vi "Display_Bad_Positions.vi"() -> ()   [LabVIEW 2022 SP3]
uses:
  Collision_Detection/Triangles/EnFlo specific/Collision Mode.ctl
  Collision_Detection/Triangles/EnFlo specific/Collision Detection global.vi
panel:
  out "Error Comments":string
  in  "Show Red Collision Sphere":bool=TRUE
  in  "Display Line Number":i32=1 min=1
  out "Table Control":string[][](table)
  in  "Choose Bad Point file":path
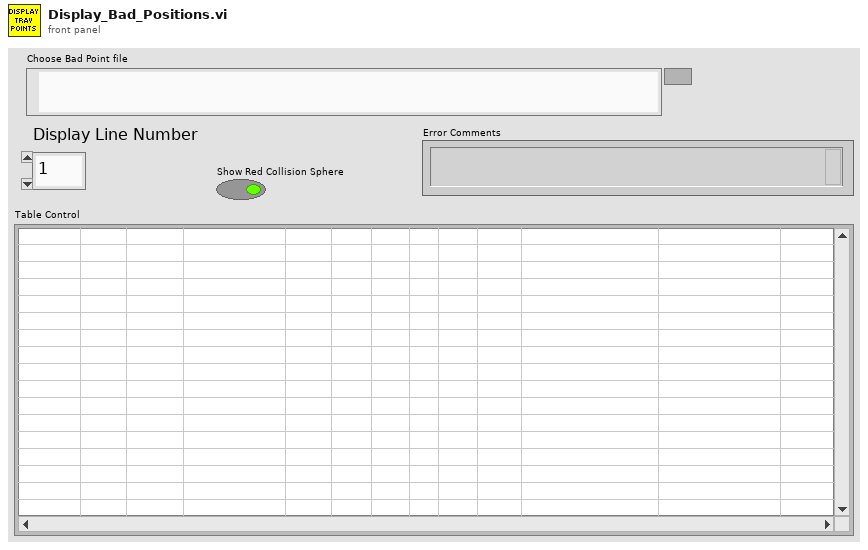
[diagram p1: front panel]
types:
  T1 = typedef "Collision Mode.ctl" = enum16{"Traverse - Tunnel", "Traverse - Model", "Traverse - Fixed objects", "Traverse - Traverse", "Traverse - All"}
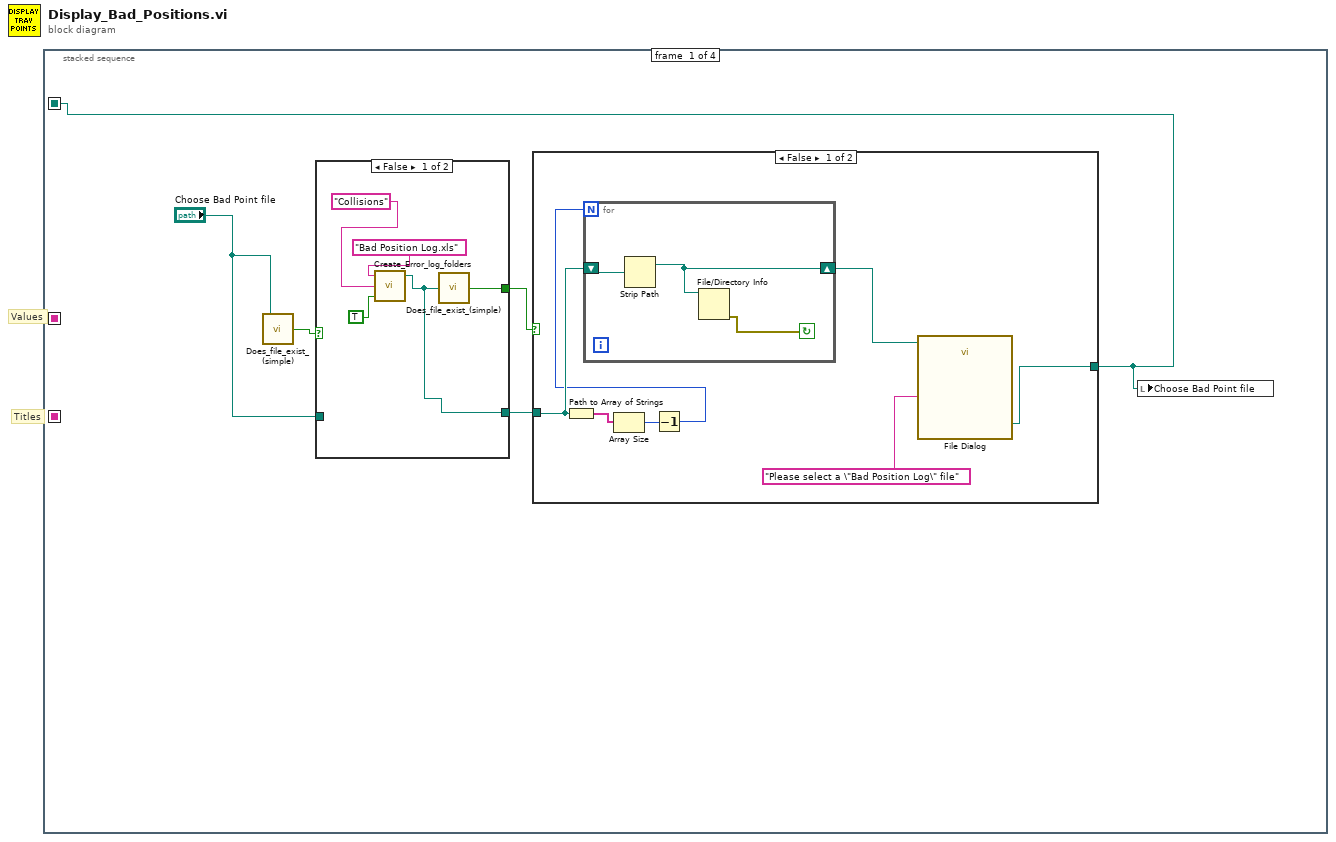
[diagram p0: block diagram]
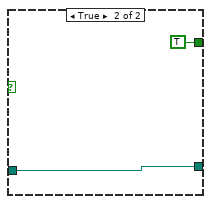
[diagram p2: hidden frame]
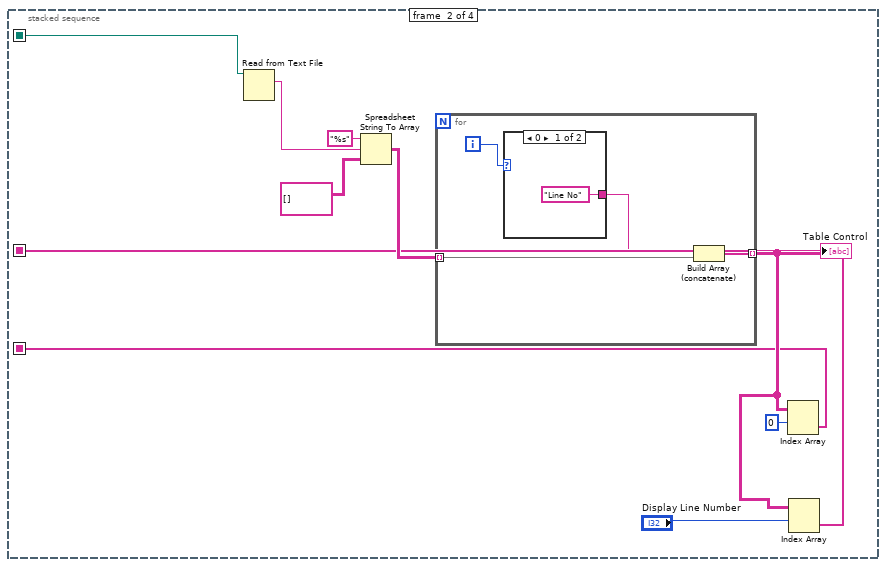
[diagram p4: hidden frame]
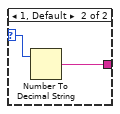
[diagram p5: hidden frame]
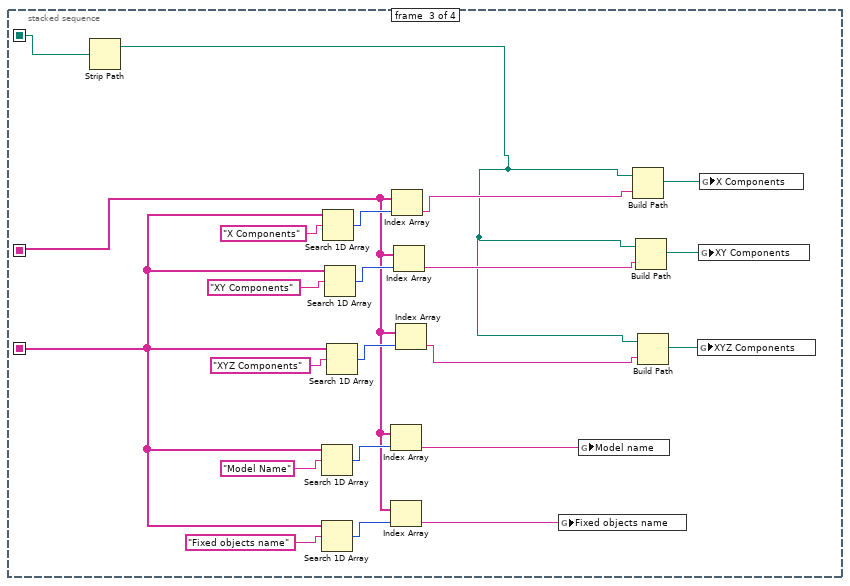
[diagram p6: hidden frame]
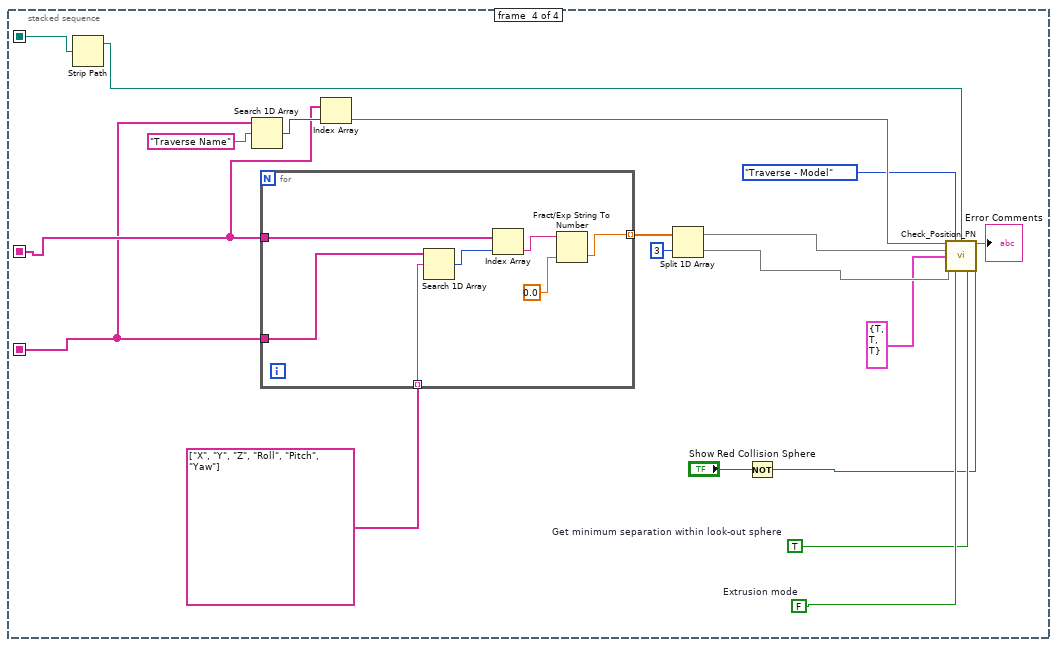
[diagram p7: hidden frame]
diagram:
  # "Values"
  # "Titles"
  n1 = stacked-sequence {
    seq-local: [_ w25 _ _] -> [_ _ w45 w75]
    seq-local: [_ w26 _ _] -> [_ _ w46 w76]
    seq-local: [w1 _ _ _] -> [_ w24 w42 w65]
    frame #0 {
      n2 = call "Does_file_exist_(simple).vi"("Pathname"="Choose Bad Point file") -> ("exists?"=w5:bool)
      n3 = case shown="False" w5 {
        tunnel: [w8 TRUE ("exists?")] -> w4
        tunnel: [w7 w12] -> w3
        tunnel: "Choose Bad Point file" -> [_ w12]
        frame False {
          n4 = call "Create_Error_log_folders.vi"("Log Filename"="Bad Position Log.xls", "Log Folder"="Collisions", "Per Day Log File?"=TRUE) -> ("Local Log File"=w7:path)  [unwired: 3 in, 1 out]
          n5 = call "Does_file_exist_(simple).vi"("Pathname"=w7) -> ("exists?"=w8:bool)
        }
        frame True {
        }
      }
      n6 = case shown="False" w4 {
        tunnel: [w18 w23] -> w1
        tunnel: w3 -> [w16 w23]
        frame False {
          n7 = Path to Array of Strings(0:w16) -> (2:w17:string[])  [unwired: 1 out]
          n8 = Array Size(array=w17) -> (size(s)=w15:i32)
          n9 = Decrement(x=w15) -> (x-1=w13:i32)
          n10 = for {
            N: w13 -> [_]
            shift-right: [w21] -> w14
            shift-left: w16 -> [w22]
            stop <- w20 continue-if-true
            n11 = Strip Path(path=w22) -> (stripped path=w21:path)  [unwired: 1 out]
            n12 = File/Directory Info(path=w21) -> (error out=w20:errorcluster)  [unwired: 1 in, 6 out]
          }
          n13 = call "File Dialog"("start path"=w14, "prompt"="Please select a \"Bad Position Log\" file") -> ("selected path"=w18:path)  [unwired: 10 in, 3 out]
        }
        frame True {
        }
      }
      n14 = local write "Choose Bad Point file"(w1) -> ()
    }
    frame #1 {
      n15 = Read from Text File(file (use dialog)=w24) -> (text=w33:string)  [unwired: 3 in, 3 out]
      n16 = Spreadsheet String To Array(format string="%s", spreadsheet string=w33, array type (2D Dbl)=string[][] []) -> (array=w30:string[][])  [unwired: 1 in]
      n17 = for {
        tunnel: w30 -> [w36] mode=indexing
        tunnel: [w35] -> w27 mode=indexing
        i -> [w34]
        n18 = case shown="0" w34 {
          selector: w34 -> [_ w39]
          tunnel: ["Line No" w40] -> w37
          frame 0 {
          }
          frame 1, Default {
            n19 = Number To Decimal String(number=w39) -> (decimal integer string=w40:string)  [unwired: 1 in]
          }
        }
        n20 = Build Array (concatenate)(w37, w36) -> (w35:string[])
      }
      "Table Control" <- w27
      n21 = Index Array(array=w27, index (row)=0) -> (element=w25:string[])  [unwired: 1 in]
      n22 = Index Array(array=w27, index (row)="Display Line Number") -> (element=w26:string[])  [unwired: 1 in]
    }
    frame #2 {
      n23 = Strip Path(path=w42) -> (stripped path=w41:path)  [unwired: 1 out]
      n24 = Search 1D Array(1D array=w45, element="Model Name" ("Error String")) -> (index of element=w52:i32)  [unwired: 1 in]
      n25 = Search 1D Array(1D array=w45, element="Fixed objects name" ("Error String")) -> (index of element=w49:i32)  [unwired: 1 in]
      n26 = Search 1D Array(1D array=w45, element="X Components" ("Error String")) -> (index of element=w58:i32)  [unwired: 1 in]
      n27 = Search 1D Array(1D array=w45, element="XY Components" ("Error String")) -> (index of element=w56:i32)  [unwired: 1 in]
      n28 = Search 1D Array(1D array=w45, element="XYZ Components" ("Error String")) -> (index of element=w53:i32)  [unwired: 1 in]
      n29 = Index Array(array=w46, index=w52) -> (element=w44:string)
      n30 = Index Array(array=w46, index=w49) -> (element=w43:string)
      n31 = Index Array(array=w46, index=w58) -> (element=w57:string)
      n32 = Index Array(array=w46, index=w56) -> (element=w47:string)
      n33 = Index Array(array=w46, index=w53) -> (element=w48:string)
      n34 = global write "Collision Detection global.vi" "Fixed objects name"(w43) -> ()
      n35 = global write "Collision Detection global.vi" "Model name"(w44) -> ()
      n36 = Build Path(base path=w41, name or relative path=w57) -> (appended path=w60:path)
      n37 = Build Path(base path=w41, name or relative path=w47) -> (appended path=w61:path)
      n38 = Build Path(base path=w41, name or relative path=w48) -> (appended path=w62:path)
      n39 = global write "Collision Detection global.vi" "XYZ Components"(w62) -> ()
      n40 = global write "Collision Detection global.vi" "XY Components"(w61) -> ()
      n41 = global write "Collision Detection global.vi" "X Components"(w60) -> ()
    }
    frame #3 {
      w70 = TRUE  # Get minimum separation within look-out sphere
      w71 = FALSE  # Extrusion mode
      n42 = Strip Path(path=w65) -> (stripped path=w64:path)  [unwired: 1 out]
      n43 = Search 1D Array(1D array=w75, element="Traverse Name" ("Error String")) -> (index of element=w78:i32)  [unwired: 1 in]
      n44 = for {
        tunnel: w75 -> [w87]
        tunnel: string[] ["X", "Y", "Z", "Roll", "Pitch", "Yaw"] ("appended array") -> [w86] mode=indexing
        tunnel: w76 -> [w85]
        tunnel: [w82] -> w80 mode=indexing
        n45 = Search 1D Array(1D array=w87, element=w86) -> (index of element=w88:i32)  [unwired: 1 in]
        n46 = Index Array(array=w85, index=w88) -> (element=w84:string)
        n47 = Fract/Exp String To Number(string=w84, default (0 dbl)=sgl 0.0 ("default (0 DBL)")) -> (number=w82:sgl)  [unwired: 2 in, 1 out]
      }
      n48 = Index Array(array=w76, index=w78) -> (element=w74:string)
      n49 = Split 1D Array(array=w80, index=3) -> (first subarray=w73:sgl[], second subarray=w72:sgl[])
      n50 = Not(x="Show Red Collision Sphere") -> (.not. x?=w66:bool)
      n51 = call "Check_Position_PN.vi"("Traverse Name"=w74, "Collision mode"=Collision_Mode."Traverse - Model", "Collision_detection"=w64, "Position to check"=w73, "Traverse Active Parts"=cluster{"X":bool, "XY":bool, "XYZ":bool} {"X"=TRUE, "XY"=TRUE, "XYZ"=TRUE}, "Model Rotation (deg)"=w72, "Extrusion mode"=w71, "Get minimum separation within look-out sphere"=w70, "Visualisation only (no collision detection)"=w66) -> ("Error Comments"=→"Error Comments":string)  [unwired: 2 in, 4 out]
    }
  }
